vi "tcs_getEvent_Heartbeat.vi"(8 "error in (no error)":errorcluster, 11 "logevent_Heartbeat_Ctl":T1) -> (0 "error out":errorcluster, 2 "function return":i32, 3 "logevent_Heartbeat_Ctl out":T1)   [LabVIEW 2016, in "SALLV_tcs.lvlib"]
doc: "int tcs_shm_getEvent_HeartbeatLV(tcs_logevent_HeartbeatLV *logevent_Heartbeat_Ctl );"
uses:
  SALLV_tcs.lvlib
  DataTypes/logevent_Heartbeat.ctl
  SALLV_tcs.so
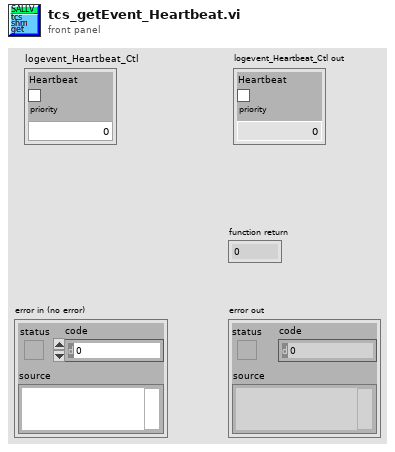
[diagram p1: front panel]
types:
  T1 = typedef "SALLV_tcs.lvlib/logevent_Heartbeat.ctl" = cluster{"Heartbeat":bool, "priority":i32}
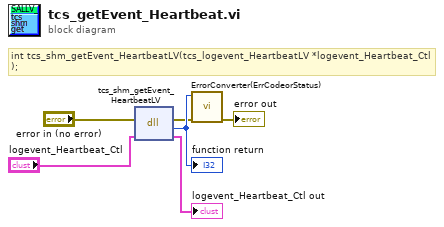
[diagram p0: block diagram]
diagram:
  # "int tcs_shm_getEvent_HeartbeatLV(tcs_logevent_HeartbeatLV *logevent_Heartbeat_Ctl );"
  n1 = dll-call lib="home/andres/Desktop/SALLV_tcs/SALLV_tcs.*" fn="tcs_shm_getEvent_HeartbeatLV"(error in="error in (no error)", "logevent_Heartbeat_Ctl"="logevent_Heartbeat_Ctl") -> (error out=w2:errorcluster, w6:i32, "logevent_Heartbeat_Ctl"=→"logevent_Heartbeat_Ctl out":T1)  [unwired: 2 in, 1 out]
  "function return" <- w6
  n2 = call "ErrorConverter(ErrCodeorStatus).vi"("error in (no error)"=w2, "error code"=w6) -> ("error out"=→"error out":errorcluster)  [unwired: 9 in]
